vi "Final Calculations.vi"() -> ()   [LabVIEW 2013]
uses:
  <vilib>/Utility/file.llb/Read From Spreadsheet File (string).vi
panel:
  out "subarray":string[][](array[string])
  out "Array":dbl[](array[numeric])
  out "String":string
  out "index of element":i32
  out "Gallons Dispensed":dbl[](array[numeric])
  out "all rows":string[][](array[string])
  in  "file path (dialog if empty)":path
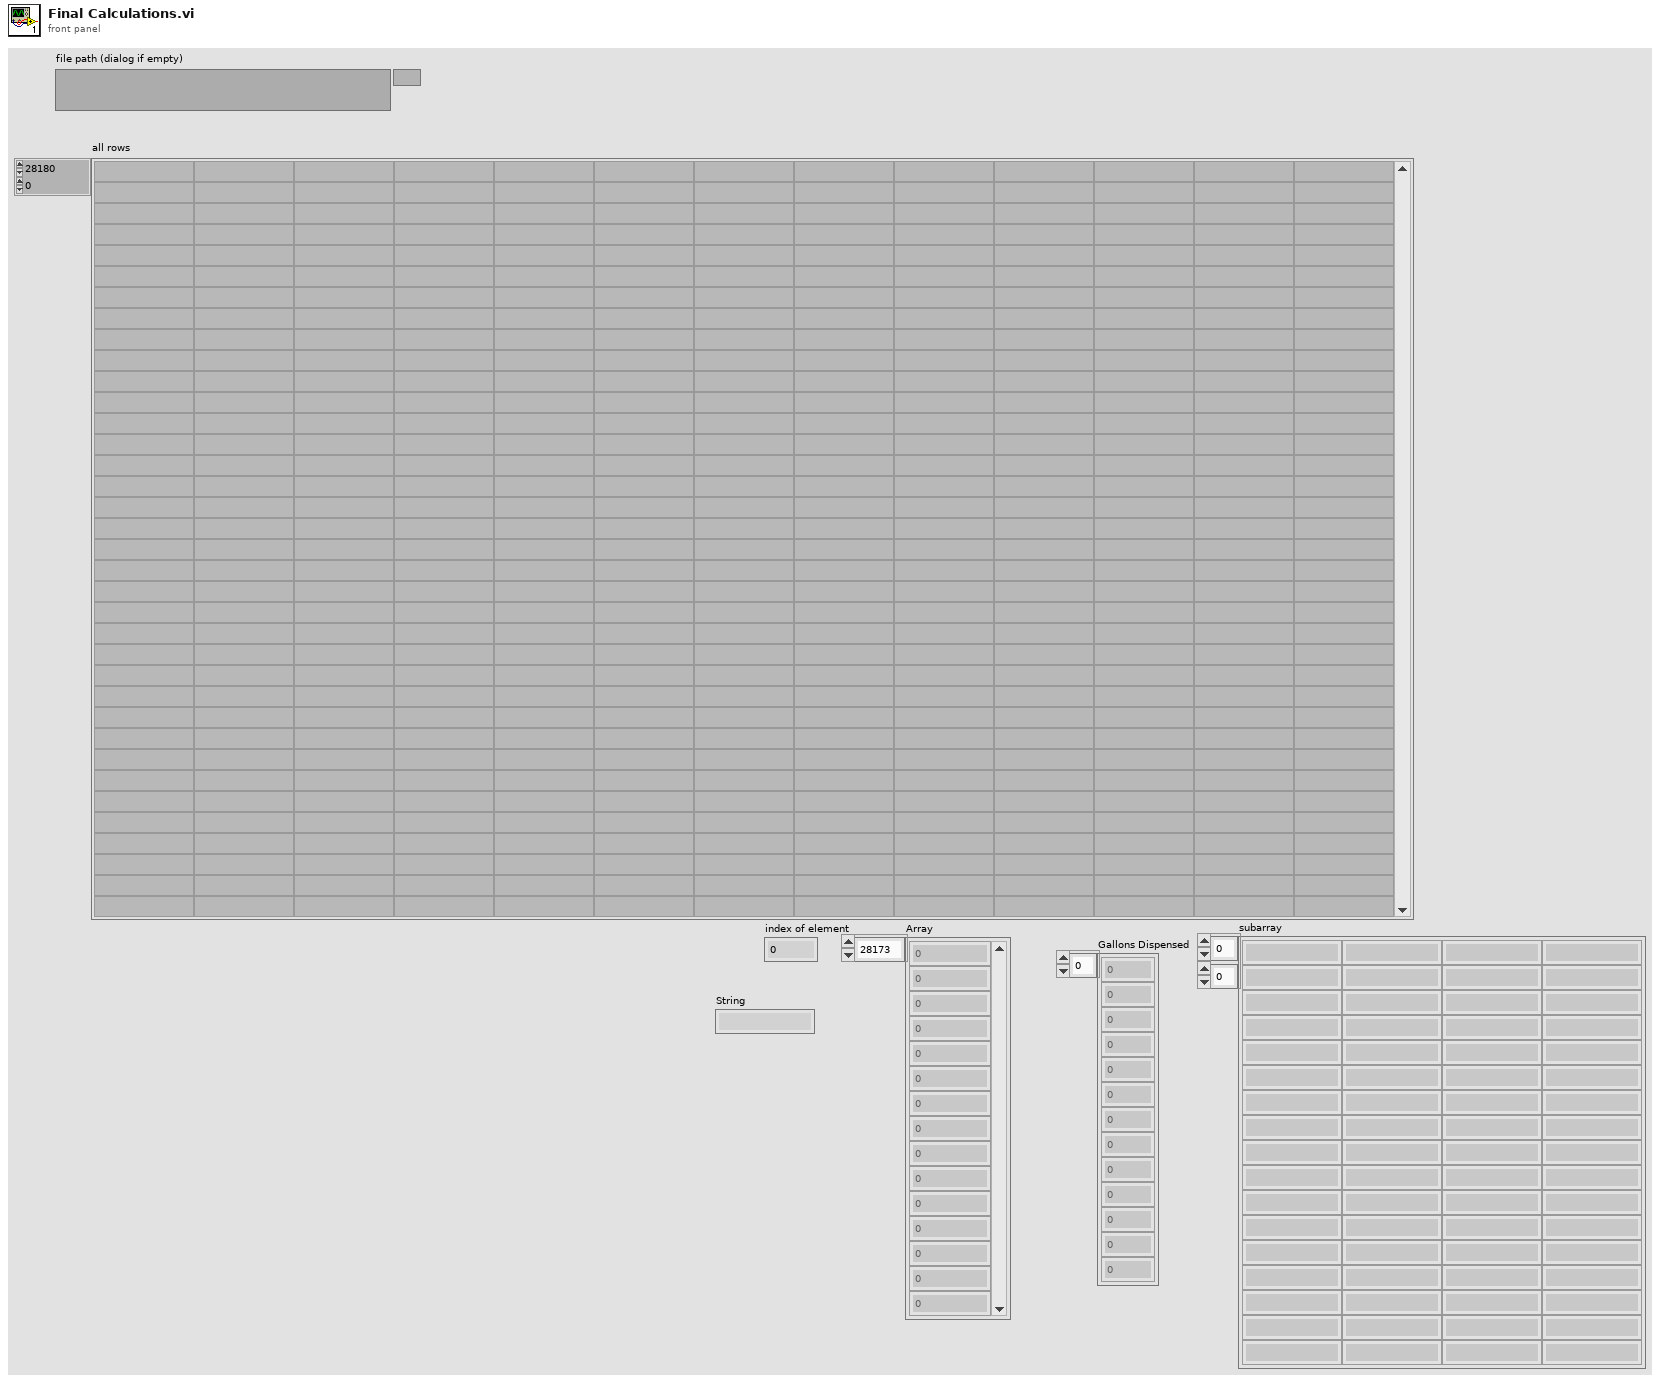
[diagram p1: front panel]
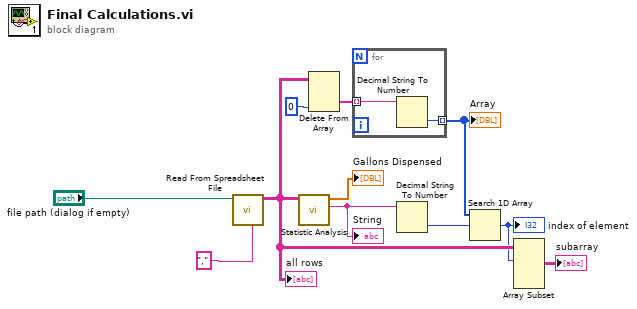
[diagram p0: block diagram]
diagram:
  n1 = call-poly <vilib>:"Read From Spreadsheet File.vi"("delimiter (\\t)"="," ("delimiter (\\t)"), "file path (dialog if empty)"="file path (dialog if empty)") -> ("all rows"=w3:string[][])  [unwired: 5 in, 4 out]
  "all rows" <- w3
  n2 = call "Statistic Analysis.vi"("All Data"=w3) -> ("String"=w5:string, "Dispensed Gallons"=→"Gallons Dispensed":dbl[])  [unwired: 9 in]
  "String" <- w5
  n3 = Delete From Array(array=w3, index (col)=0 ("disabled index (col)")) -> (deleted portion=w6:string[])  [unwired: 2 in, 1 out]
  n4 = for {
    tunnel: w6 -> [w13] mode=indexing
    tunnel: [w12] -> w7 mode=indexing
    n5 = Decimal String To Number(string=w13) -> (number=w12:i32)  [unwired: 2 in, 1 out]
  }
  "Array" <- w7
  n6 = Decimal String To Number(string=w5) -> (number=w4:i32)  [unwired: 2 in, 1 out]
  n7 = Search 1D Array(1D array=w7, element=w4) -> (index of element=w2:i32)  [unwired: 1 in]
  "index of element" <- w2
  n8 = Array Subset(array=w3, index (row)=w2) -> (→"subarray":string[][])  [unwired: 3 in]
